vi "Match Unit.vi"(8 "error in (no error)":errorcluster, 10 "Unit Read":string, 11 "BH Druck PACE Series in":refnum<class "BH Druck PACE Series.lvclass">) -> (0 "error out":errorcluster, 2 "Unit Display":string, 3 "BH Druck PACE Series out":refnum<class "BH Druck PACE Series.lvclass">)   [LabVIEW 2022 SP3, in "BH Druck PACE Series.lvclass"]
uses:
  BH Druck PACE Series.lvclass
  BH Druck PACE Series.lvclass/BH Druck PACE Series.ctl
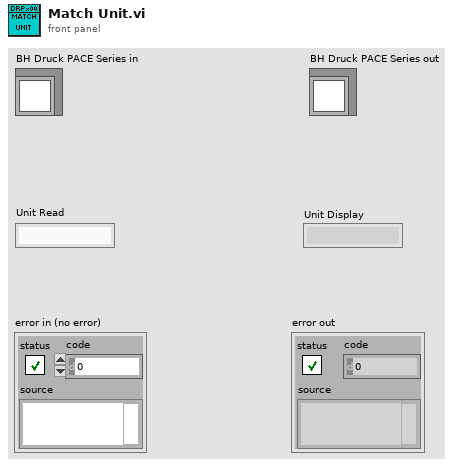
[diagram p1: front panel]
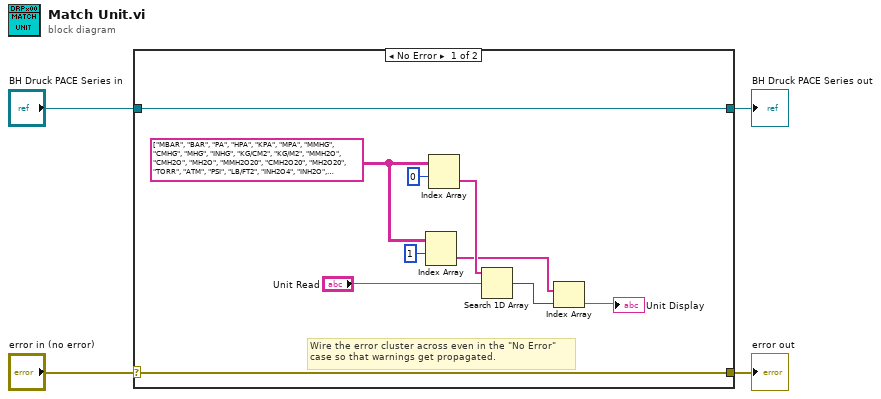
[diagram p0: block diagram]
diagram:
  n1 = case shown="No Error" "error in (no error)" {
    selector: "error in (no error)" -> [w13 w16]
    tunnel: [w13 w16] -> w3
    tunnel: [w14 w15] -> w1
    tunnel: "BH Druck PACE Series in" -> [w14 w15]
    frame No Error {
      w9 = string[][] [["MBAR", "BAR", "PA", "HPA", "KPA", "MPA", "MMHG", "CMHG", "MHG", "INHG", "KG/CM2", "KG/M2", "MMH2O", "CMH2O", "MH2O", "MMH2O20", "CMH2O20", "MH2O20", "TORR", "ATM", "PSI", "LB/FT2", "INH2O4", "INH2O", "INH2O60", "FTH2O4", "FTH2O", "FTH2O60", "USER1", "USER2", "USER3", "USER4"], ["mbar", "bar", "Pa", "hPa", "kPa", "mPa", "mmHg@0°C", "cmHg@0°C", "mHg@0°C", "inHg@0°C", "kg/cm2", "kg/m2", "mmH2O@4°C", "cmH2O@4°C", "mH2O@4°C", "mmH2O@20°C", "cmH2O@20°C", "mH2O@20°C", "torr", "atm", "psi", "lb/ft2", "inH2O@4°C", "inH2O@20°C", "inH2O@60°F", "ftH2O@4°C", "ftH2O@20°C", "ftH2O@60°F", "UserUnit1", "UserUnit2", "UserUnit3", "UserUnit4"]]
      # "Wire the error cluster across even in the \"No Error\"\ncase so that warnings get propagated."
      n2 = Index Array(array=w9, index (row)=1) -> (element=w6:string[])  [unwired: 1 in]
      n3 = Index Array(array=w9, index (row)=0) -> (element=w8:string[])  [unwired: 1 in]
      n4 = Search 1D Array(1D array=w8, element="Unit Read") -> (index of element=w7:i32)  [unwired: 1 in]
      n5 = Index Array(array=w6, index=w7) -> (element=→"Unit Display":string)
    }
    frame Error {
    }
  }
  "error out" <- w3
  "BH Druck PACE Series out" <- w1
